vi "Read Sub Panel.vi"(8 "error in (no error)":errorcluster, 11 "SubPanel.lvclass in":refnum<class "SubPanel.lvclass">) -> (0 "error out":errorcluster, 2 "Sub Panel":refnum<vi>, 3 "SubPanel.lvclass out":refnum<class "SubPanel.lvclass">)   [LabVIEW 2012, in "SubPanel.lvlib" / "SubPanel.lvclass"]
uses:
  SubPanel.lvclass
  SubPanel.lvclass/SubPanel.ctl
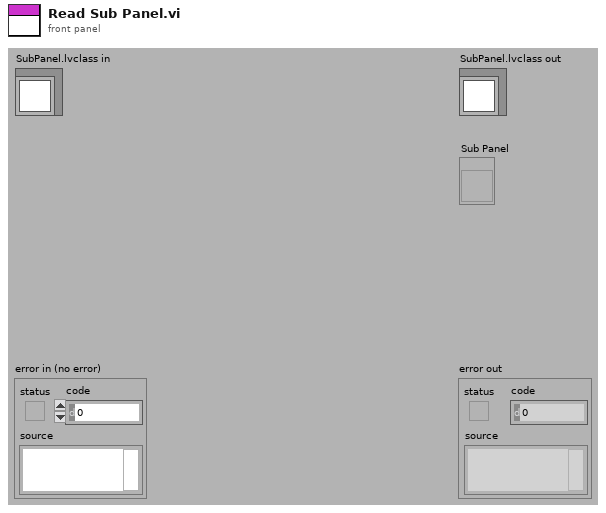
[diagram p1: front panel]
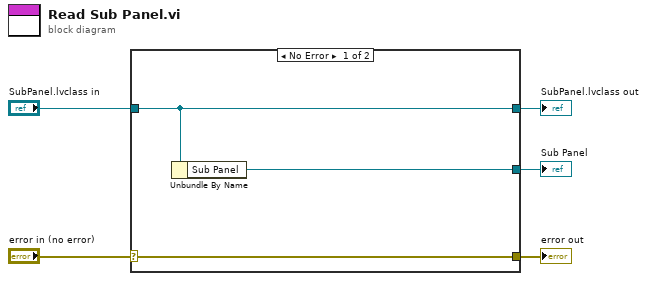
[diagram p0: block diagram]
diagram:
  n1 = case shown="No Error" "error in (no error)" {
    selector: "error in (no error)" -> [w8 w9]
    tunnel: [w8 w9] -> w4
    tunnel: [w7 w10] -> w2
    tunnel: "SubPanel.lvclass in" -> [w7 w10]
    tunnel: [w6 _] -> w1
    frame No Error {
      n2 = Unbundle By Name(w7) -> ("Sub Panel"=w6:refnum<vi>)
    }
    frame Error {
    }
  }
  "error out" <- w4
  "SubPanel.lvclass out" <- w2
  "Sub Panel" <- w1
